vi "PRACTICA 4  PDS.vi"() -> ()   [LabVIEW 2015]
uses:
  <vilib>/MakerHub/LINX/Public/Peripherals/PWM/PWM Set Duty Cycle 1 Chan.vi
  <vilib>/MakerHub/LINX/Public/Peripherals/Analog/Analog Read 1 Chan.vi
  <vilib>/MakerHub/LINX/Public/Peripherals/Analog/Analog Read N Chans.vi
  <vilib>/MakerHub/LINX/Private/Local IO/LinxAnalogRead.vi
  <vilib>/MakerHub/LINX/Public/Utilities/Check Channel.vi
  <vilib>/MakerHub/LINX/Public/Utilities/Open Serial.vi
  <vilib>/Utility/file.llb/Write Delimited Spreadsheet (DBL).vi
  <vilib>/MakerHub/LINX/Public/Peripherals/PWM/PWM Set Duty Cycle N Chans.vi
  <vilib>/MakerHub/LINX/Private/Utilties/Generate Error.vi
  <vilib>/MakerHub/LINX/LMH-LINX.lvlib
panel:
  in  "?":bool
  in  "Serial Port 2":refnum<visa-resource-name>
  out "XY Graph":cluster{dbl[], dbl[]}(graph)
  out "Analog Data":dbl
  out "XY Graph 2":cluster{dbl[], dbl[]}(graph)
  in  "?":bool
  out "Loop Rate (Hz)":u32
  in  "Analog Channel":u8
  in  "DO Output Channel":u8
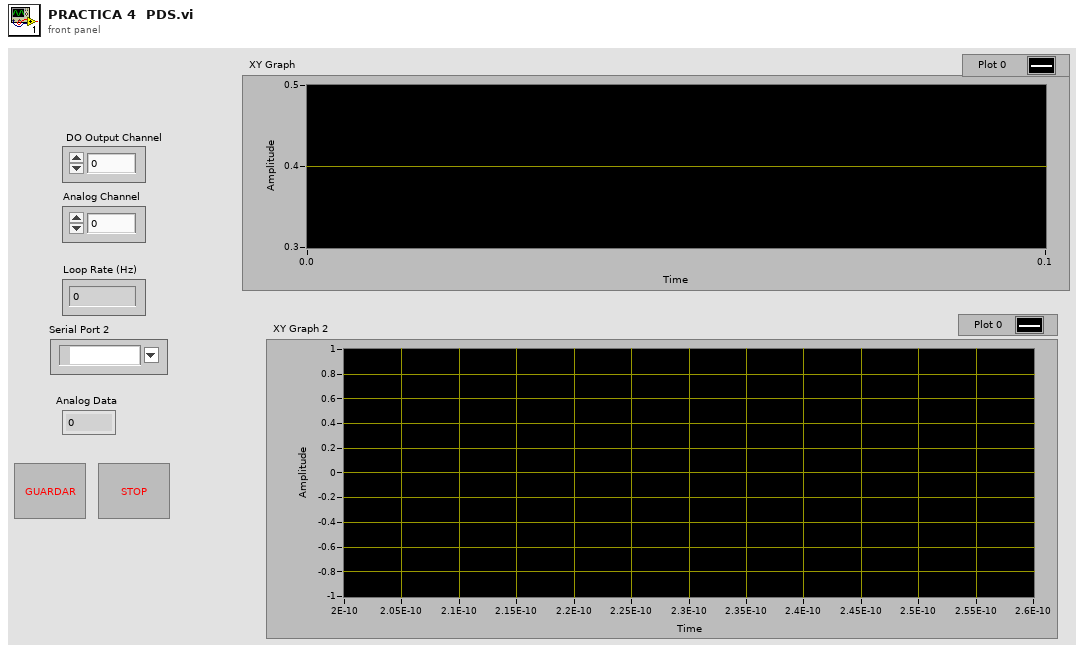
[diagram p1: front panel]
types:
  T1 = typedef "LMH-LINX.lvlib/LINX Ref.ctl" = cluster{"IO":T2, "Interface":T3, "LINX Device Config":T4}
  T2 = typedef "LMH-LINX.lvlib/Platform.ctl" = enum16{"Remote", "Local"}
  T3 = typedef "LMH-LINX.lvlib/Interface.ctl" = enum16{"Serial", "TCP"}
  T4 = typedef "LMH-LINX.lvlib/Device.lvlib/LINX Device Config.ctl" = cluster{"Interface":T3, "COM Port":refnum<visa-resource-name>, "TCP Configuration":T5, "Device Family":u8, "Device ID":u8, "Device Name":string, "TCP Ref":refnum<k5>, "Channels":T6}
  T5 = typedef "LMH-LINX.lvlib/Device.lvlib/TCP Config.ctl" = cluster{"IP Address":string, "Port":u16}
  T6 = typedef "LMH-LINX.lvlib/Channels.ctl" = cluster{"DI":u8[], "DO":u8[], "AI":u8[], "AO":u8[], "PWM":u8[], "QE":u8[], "UART":u8[], "I2C 2":u8[], "SPI":u8[], "CAN":u8[], "Servo":u8[], "AI Ref (V)":dbl, "AI Resolution (Bits)":u8, "AO Ref (V)":dbl, "AO Resolution (Bits)":u8}
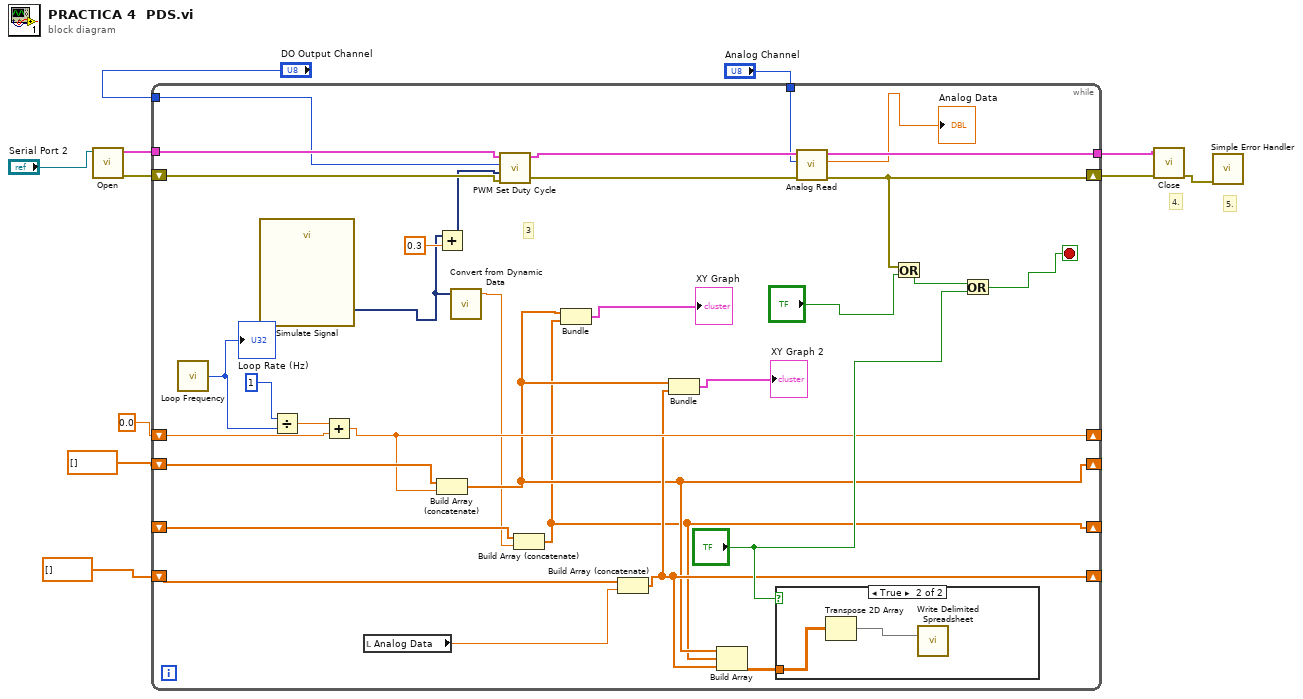
[diagram p0: block diagram]
diagram:
  # "5."
  # "4."
  n1 = call-poly <vilib>:"Open.vi"("Serial Port"="Serial Port 2") -> ("Error Out"=w10:errorcluster, "LINX Resource"=w11:T1)  [unwired: 8 in, 1 out]
  n2 = while {
    tunnel: w11 -> [w43]
    tunnel: [w39] -> w9
    tunnel: "DO Output Channel" -> [w38]
    tunnel: "Analog Channel" -> [w37]
    shift-right: [w36] -> w8
    shift-left: w10 -> [w42]
    shift-right: [w28] -> _
    shift-left: 0.0 ("y") -> [w32]
    shift-right: [w23] -> _
    shift-left: dbl[] [] ("Numeric") -> [w29]
    shift-right: [w24] -> _
    shift-left: dbl[] [] ("element") -> [w27]
    shift-right: [w18] -> _
    shift-left: _ -> [w20]
    stop <- w35 stop-if-true
    # "3"
    n3 = call <vilib>:"Loop Frequency.vi"() -> ("Loop Rate (Hz)"=w17:u32)
    "Loop Rate (Hz)" <- w17
    n4 = call "Simulate Signal"() -> ("Square"=w13:dynamicdata)  [unwired: 14 in, 1 out]
    n5 = Divide(x=u32 1 ("Loop Rate (Hz)"), y=w17) -> (x/y=w33:dbl)
    n6 = Add(x=w33, y=w32) -> (x+y=w28:dbl)
    n7 = local read "Analog Data"() -> (w26:dbl)
    n8 = Add(x=w13, y=0.3) -> (x+y=w12:dynamicdata)
    n9 = Build Array (concatenate)(w29, w28) -> (w23:dbl[])
    n10 = call "Convert from Dynamic Data"("Dynamic Data Type"=w13) -> ("Scalar"=w19:dbl)  [unwired: 3 in]
    n11 = call-poly <vilib>:"PWM Set Duty Cycle.vi"("Error In"=w42, "Duty Cycle (0-1)"=w12, "PWM Channel"=w38, "LINX Resource"=w43) -> ("Error Out"=w40:errorcluster, "LINX Resource"=w41:T1)  [unwired: 6 in]
    n12 = Build Array (concatenate)(w20, w19) -> (w18:dbl[])
    n13 = Bundle(w23, w18) -> (→"XY Graph":cluster{dbl[], dbl[]})  [unwired: 1 in]
    n14 = Build Array (concatenate)(w27, w26) -> (w24:dbl[])
    n15 = Bundle(w23, w24) -> (→"XY Graph 2":cluster{dbl[], dbl[]})  [unwired: 1 in]
    n16 = Build Array(w23, w18, w24) -> (w22:dbl[][])
    n17 = case shown="True" "?" {
      tunnel: w22 -> [_ w45]
      frame False {
      }
      frame True {
        n18 = Transpose 2D Array(2D array=w45) -> (transposed array=w44:dbl[][])
        n19 = call-poly <vilib>:"Write Delimited Spreadsheet.vi"("2D data"=w44) -> ()  [unwired: 13 in, 2 out]
      }
    }
    n20 = call-poly <vilib>:"Analog Read.vi"("Error In"=w40, "Analog Channel"=w37, "LINX Resource"=w41) -> ("Error Out"=w36:errorcluster, "Voltage"=→"Analog Data":dbl, "LINX Resource"=w39:T1)  [unwired: 5 in, 1 out]
    n21 = Or(x=w36, y="?") -> (x .or. y?=w34:bool)
    n22 = Or(x=w34, y="?") -> (x .or. y?=w35:bool)
  }
  n23 = call <vilib>:"Close.vi"("Error In"=w8, "LINX Resource"=w9) -> ("Error Out"=w7:errorcluster)  [unwired: 9 in]
  n24 = call <vilib>:"Simple Error Handler.vi"("error in (no error)"=w7) -> ()  [unwired: 4 in, 5 out]
